vi "Get exp param.vi"(8 "error in (no error)":errorcluster, 11 "Experiment in":refnum<class "Experiment.lvclass">) -> (0 "error out":errorcluster, 1 "WCM_correction":bool, 2 "All":bool, 3 "Experiment out":refnum<class "Experiment.lvclass">, 5 "#pp":i32)   [LabVIEW 2018, in "Experiment.lvclass"]
uses:
  Experiment.lvclass
  Experiment.lvclass/Experiment.ctl
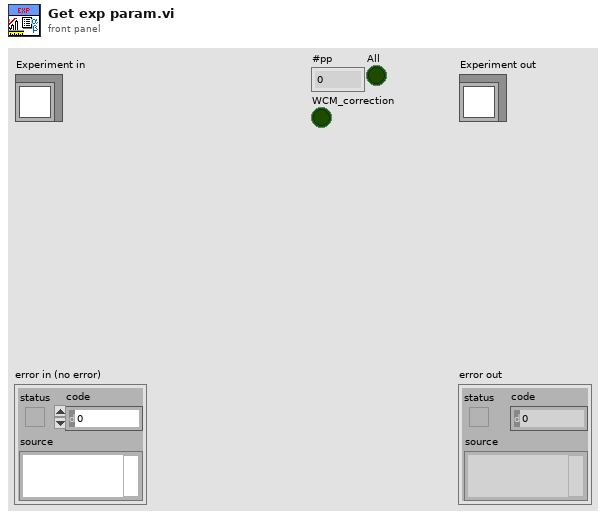
[diagram p1: front panel]
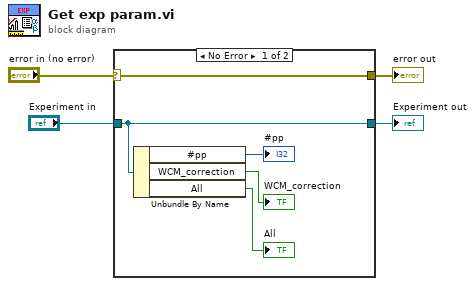
[diagram p0: block diagram]
diagram:
  n1 = case shown="No Error" "error in (no error)" {
    selector: "error in (no error)" -> [w9 w11]
    tunnel: [w9 w11] -> w3
    tunnel: [w8 w10] -> w1
    tunnel: "Experiment in" -> [w8 w10]
    frame No Error {
      n2 = Unbundle By Name(w8) -> ("#pp"=→"#pp":i32, "WCM_correction"=→"WCM_correction":bool, "All"=→"All":bool)
    }
    frame Error {
    }
  }
  "error out" <- w3
  "Experiment out" <- w1
